vi "UserElapsedTIme.vi"() -> ()   [LabVIEW 2020]
panel:
  out "TimeElapsed?":bool
  in  "TimeTarget":dbl
  in  "Reset?":bool
  in  "stop":bool
  out "ElpasedTime":dbl
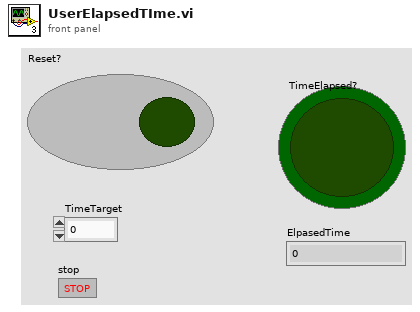
[diagram p1: front panel]
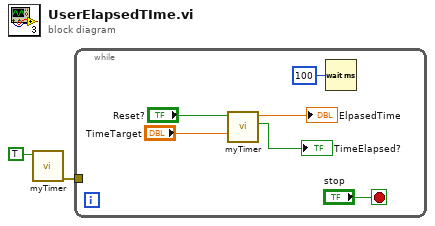
[diagram p0: block diagram]
diagram:
  n1 = call "myTimer.vi"("Reset?"=TRUE) -> ("error out"=w2:errorcluster)  [unwired: 8 in, 2 out]
  n2 = while {
    tunnel: w2 -> [_]
    stop <- "stop" stop-if-true
    n3 = call "myTimer.vi"("TimeTarget"="TimeTarget", "Reset?"="Reset?") -> ("TimeElapsed?"=→"TimeElapsed?":bool, "ElpasedTime"=→"ElpasedTime":dbl)  [unwired: 7 in, 1 out]
    n4 = Wait (ms)(milliseconds to wait=u32 100) -> ()  [unwired: 1 out]
  }
